vi "Matt-Vibrometer.vi"() -> ()   [LabVIEW 2016]
uses:
  VIs/uPythonX/uPythonX.xctl
panel:
  in  "Tab Control":T1(tab)=enum."Class"
  in  "Vibrometer":T2(xcontrol)={"VISA Refnum in"="ASRL93::INSTR", "Python Code"="import Bars,ssd1327\n\nimport VibSerial\nfrom machine import I2C, Pin\nfrom pyb import ADC  # ADC on machine is limited to under 1.7V\n\ni2c = I2C(2)  # screen\nuart = pyb.UART(1,9600, bits=8, parity=None, stop=1) # vibrometer\ndisplay = ssd1327.SEEED_OLED_96X96(i2c)   # set up display\ndisplay.fill(0)\nlights = Bars.GroveLEDBar('W32','W30',False)\nadc = ADC('X1')\n\n# initialize vibrometer\nsettings = VibSerial.setup(104, 50, True, True)  \nprint(settings)\nSettings = settings.split(', ')\n\n# show settings\ndisplay.text(\"Matt's Box\",0,0,15)\ndisplay.text(' ',0,10,5)\ndisplay.text('HP ' + Settings[0] + 'Hz',0,20,15)\ndisplay.text('BW ' + Settings[1] + 'kHz',0,30,15)\ndisplay.text('S ' + Settings[2] + ' mmps',0,40,15)\ndisplay.show()\n\nwhile True:\n     lights.meter(int(adc.read()/4095*11))\n     utime.sleep(.2)\n     \n"}
  in  "VibSerial":T2(xcontrol)={"VISA Refnum in"="ASRL93::INSTR", "Python Code"="Answer = b'AgAAAAAAAAAAAAAAAAAGAAAAAio=\\n'\n\n#  Laser Toggle\nLaserOn = 'AQAAAAAAAAAAAAAAAAAQAAAAAAAEAgAuAAEAAwEA\\n'\nLaserOff = 'AQAAAAAAAAAAAAAAAAAQAAAAAAAEAgAuAAEAAwAA\\n'\n\n# High Pass Filter\nHighPass_Off = 'AQAAAAAAAAAAAAAAAAAQAAAAAAAEBwAuAgEAAwAA\\n'\nHighPass_13Hz = 'AQAAAAAAAAAAAAAAAAAQAAAAAAAEBwAuAgEAAwEA\\n'\nHighPass_104Hz = 'AQAAAAAAAAAAAAAAAAAQAAAAAAAEBwAuAgEAAwIA\\n'\n\n# Bandwidth\nBandwidth_1kHz = 'AQAAAAAAAAAAAAAAAAAQAAAAAAAEBwASAAEAAwUA\\n'\nBandwidth_5kHz = 'AQAAAAAAAAAAAAAAAAAQAAAAAAAEBwASAAEAAwQA\\n'\nBandwidth_10kHz = 'AQAAAAAAAAAAAAAAAAAQAAAAAAAEBwASAAEAAwMA\\n'\nBandwidth_25kHz = 'AQAAAAAAAAAAAAAAAAAQAAAAAAAEBwASAAEAAwIA\\n'\nBandwidth_50kHz = 'AQAAAAAAAAAAAAAAAAAQAAAAAAAEBwASAAEAAwEA\\n'\nBandwidth_100kHz = 'AQAAAAAAAAAAAAAAAAAQAAAAAAAEBwASAAEAAwAA\\n'\n\n# Sensitivity\nSensitivity_10mmps = 'AQAAAAAAAAAAAAAAAAAQAAAAAAAEBwAKAAEAAwcA\\n'\nSensitivity_20mmps = 'AQAAAAAAAAAAAAAAAAAQAAAAAAAEBwAKAAEAAwYA\\n'\nSensitivity_50mmps = 'AQAAAAAAAAAAAAAAAAAQAAAAAAAEBwAKAAEAAwUA\\n'\nSensitivity_100mmps = 'AQAAAAAAAAAAAAAAAAAQAAAAAAAEBwAKAAEAAwQA\\n'\nSensitivity_200mmps = 'AQAAAAAAAAAAAAAAAAAQAAAAAAAEBwAKAAEAAwMA\\n'\nSensitivity_500mmps = 'AQAAAAAAAAAAAAAAAAAQAAAAAAAEBwAKAAEAAwIA\\n'\nSensitivity_1000mmps = 'AQAAAAAAAAAAAAAAAAAQAAAAAAAEBwAKAAEAAwEA\\n'\nSensitivity_2000mmps = 'AQAAAAAAAAAAAAAAAAAQAAAAAAAEBwAKAAEAAwAA\\n'\n\n# AutoFocus\nFocus = 'AQAAAAAAAAAAAAAAAAAQAAAAAAAEAgBAAAEAAwEA\\n'\n\nlut = {'HP0' : HighPass_Off,'HP13' : HighPass_13Hz,'HP104' : HighPass_104Hz,'BW1' : Bandwidth_1kHz, 'BW5' : Bandwidth_5kHz,'BW10' : Bandwidth_10kHz,'BW25' : Bandwidth_25kHz, 'BW50' : Bandwidth_50kHz, 'BW100' : Bandwidth_100kHz, 'S10' : Sensitivity_10mmps, 'S20' : Sensitivity_20mmps, 'S50' : Sensitivity_50mmps, 'S100' : Sensitivity_100mmps, 'S200' : Sensitivity_200mmps, 'S500' : Sensitivity_500mmps, 'S1000' : Sensitivity_1000mmps, 'S2000' : Sensitivity_2000mmps}\n\ndef Laser(Cmd):  # 0... off, 1... on, 2... focus\n     if (Cmd == 2):\n          vibSet(Focus)\n     elif (Cmd == 1):\n          vibSet(LaserOn)\n     else:\n          vibSet(LaserOff)\n          \ndef vibSet(CmdString):\n     uart.write(CmdString)\n     reply = uart.readline()\n     return (reply == Answer)\n     \ndef PassThrough():\n     if uart.any():\n          uart.readline()  # need more here - need two different serial lines\n          \n\ndef setup(filter=104, bandwidth=50, sensitivity=200, On = True, focus = True):\n\n     reply = ''\n\n     # set high pass filter\n     try:\n          value = lut['HP'+str(filter)]\n     except:\n          value = lut['HP104']\n          filter = 104\n     if vibSet(value):\n          reply = reply + str(filter)\n\n     # set bandwidth\n     try:\n          value = lut['BW'+str(bandwidth)]\n     except:\n          value = lut['BW50']\n          bandwidth = 50\n     if vibSet(value):\n          reply = reply +  ', ' + str(bandwidth)\n\n     # set sensitivity\n     try:\n          value = lut['S'+str(sensitivity)]\n     except:\n          value = lut['S200']\n          sensitivity = 200\n     if vibSet(value):\n          reply = reply +  ', ' + str(sensitivity)\n\n     #turn laser on and autofocus\n     Laser(On)\n     if focus:\n          Laser(2)\n     return reply\n"}
  in  "VibSerial":T2(xcontrol)={"VISA Refnum in"="ASRL93::INSTR", "Python Code"="Answer = b'AgAAAAAAAAAAAAAAAAAGAAAAAio=\\n'\n          \n#  Laser Toggle\nLaserOn = 'AQAAAAAAAAAAAAAAAAAQAAAAAAAEAgAuAAEAAwEA\\n'\nLaserOff = 'AQAAAAAAAAAAAAAAAAAQAAAAAAAEAgAuAAEAAwAA\\n'\n          \n# High Pass Filter\nHighPass_Off = 'AQAAAAAAAAAAAAAAAAAQAAAAAAAEBwAuAgEAAwAA\\n'\nHighPass_13Hz = 'AQAAAAAAAAAAAAAAAAAQAAAAAAAEBwAuAgEAAwEA\\n'\nHighPass_104Hz = 'AQAAAAAAAAAAAAAAAAAQAAAAAAAEBwAuAgEAAwIA\\n'\n          \n# Bandwidth\nBandwidth_1kHz = 'AQAAAAAAAAAAAAAAAAAQAAAAAAAEBwASAAEAAwUA\\n'\nBandwidth_5kHz = 'AQAAAAAAAAAAAAAAAAAQAAAAAAAEBwASAAEAAwQA\\n'\nBandwidth_10kHz = 'AQAAAAAAAAAAAAAAAAAQAAAAAAAEBwASAAEAAwMA\\n'\nBandwidth_25kHz = 'AQAAAAAAAAAAAAAAAAAQAAAAAAAEBwASAAEAAwIA\\n'\nBandwidth_50kHz = 'AQAAAAAAAAAAAAAAAAAQAAAAAAAEBwASAAEAAwEA\\n'\nBandwidth_100kHz = 'AQAAAAAAAAAAAAAAAAAQAAAAAAAEBwASAAEAAwAA\\n'\n          \n# Sensitivity\nSensitivity_10mmps = 'AQAAAAAAAAAAAAAAAAAQAAAAAAAEBwAKAAEAAwcA\\n'\nSensitivity_20mmps = 'AQAAAAAAAAAAAAAAAAAQAAAAAAAEBwAKAAEAAwYA\\n'\nSensitivity_50mmps = 'AQAAAAAAAAAAAAAAAAAQAAAAAAAEBwAKAAEAAwUA\\n'\nSensitivity_100mmps = 'AQAAAAAAAAAAAAAAAAAQAAAAAAAEBwAKAAEAAwQA\\n'\nSensitivity_200mmps = 'AQAAAAAAAAAAAAAAAAAQAAAAAAAEBwAKAAEAAwMA\\n'\nSensitivity_500mmps = 'AQAAAAAAAAAAAAAAAAAQAAAAAAAEBwAKAAEAAwIA\\n'\nSensitivity_1000mmps = 'AQAAAAAAAAAAAAAAAAAQAAAAAAAEBwAKAAEAAwEA\\n'\nSensitivity_2000mmps = 'AQAAAAAAAAAAAAAAAAAQAAAAAAAEBwAKAAEAAwAA\\n'\n          \n# AutoFocus\nFocus = 'AQAAAAAAAAAAAAAAAAAQAAAAAAAEAgBAAAEAAwEA\\n'\n\nclass Vib(object):\n     def __init__(self,UIn,UOut):\n          self.lut = {'HP0' : HighPass_Off,'HP13' : HighPass_13Hz,'HP104' : HighPass_104Hz,'BW1' : Bandwidth_1kHz, 'BW5' : Bandwidth_5kHz,'BW10' : Bandwidth_10kHz,'BW25' : Bandwidth_25kHz, 'BW50' : Bandwidth_50kHz, 'BW100' : Bandwidth_100kHz, 'S10' : Sensitivity_10mmps, 'S20' : Sensitivity_20mmps, 'S50' : Sensitivity_50mmps, 'S100' : Sensitivity_100mmps, 'S200' : Sensitivity_200mmps, 'S500' : Sensitivity_500mmps, 'S1000' : Sensitivity_1000mmps, 'S2000' : Sensitivity_2000mmps}\n          self.uartIN = pyb.UART(UIn,9600, bits=8, parity=None, stop=1) # vibrometer\n          self.uartOUT = pyb.UART(UOut,9600, bits=8, parity=None, stop=1) # vibrometer\n\n     def Laser(self,Cmd):  # 0... off, 1... on, 2... focus\n          if (Cmd == 2):\n               self.vibSet(Focus)\n          elif (Cmd == 1):\n               self.vibSet(LaserOn)\n          else:\n               self.vibSet(LaserOff)\n          \n     def vibSet(self,CmdString):\n          self.uartOUT.write(CmdString)\n          reply = self.uartOUT.readline()\n          return (reply == Answer)\n     \n     def PassThrough(self):\n          if self.uartIN.any():\n               sent = self.uartIN.readline()  # need more here - need two different serial lines\n               seld.uart.OUT.write(sent)\n\n     def setup(self,filter=104, bandwidth=50, sensitivity=200, On = True, focus = True):\n\n          reply = ''\n\n          # set high pass filter\n          try:\n               value = self.lut['HP'+str(filter)]\n          except:\n               value = self.lut['HP104']\n               filter = 104\n          if self.vibSet(value):\n               reply = reply + str(filter)\n\n          # set bandwidth\n          try:\n               value = self.lut['BW'+str(bandwidth)]\n          except:\n               value = self.lut['BW50']\n               bandwidth = 50\n          if self.vibSet(value):\n               reply = reply +  ', ' + str(bandwidth)\n\n          # set sensitivity\n          try:\n               value = self.lut['S'+str(sensitivity)]\n          except:\n               value = self.lut['S200']\n               sensitivity = 200\n          if self.vibSet(value):\n               reply = reply +  ', ' + str(sensitivity)\n\n          #turn laser on and autofocus\n          self.Laser(LaserOn)\n          if focus:\n               self.Laser(2)\n          return reply\n"}
  in  "Bars":T2(xcontrol)={"VISA Refnum in"="ASRL93::INSTR", "Python Code"="'''\nhttp://wiki.seeedstudio.com/Grove-LED_Bar/\nhttps://github.com/Seeed-Studio/Grove_LED_Bar/blob/master/Grove_LED_Bar.cpp\nhttps://github.com/Seeed-Studio/Grove_LED_Bar/blob/master/examples/BasicControl/BasicControl.ino\n\nconnections: \nGround (B) - GND \nPower  (R)   - 3V3 \nDCLK (W) - pin W30\nDIn (Y) -  pin W32\n'''\n\nimport  utime\nfrom machine import Pin\n\nGLB_CMDMODE = 0x00  # Work on 8-bit mode\nMAX_BRIGHTNESS = 0xFF\n\nclass GroveLEDBar(object):\n     def __init__(self, dio,clk,RtoG=True):\n          self.dio = Pin(dio, Pin.OUT,Pin.PULL_UP)\n          self.clk = Pin(clk, Pin.OUT,Pin.PULL_UP)\n          self.RtoG = RtoG\n          self.stateArray = bytearray(10)\n          for i in range(10):\n               self.stateArray[i] = 0x00  # allows me to toggle individual elements\n\n     def sendData(self,data):\n          state = 0\n          for i in range(16):\n               state1 = (data & 0x8000)\n               self.dio.value(state1)\n               state=1-state\n               self.clk.value(state)\n               data<<=1\n          \n     def latchData(self):\n          self.dio.value(0)\n          utime.sleep_ms(10)\n          for i in range(4):\n               self.dio.value(1)\n               utime.sleep_us(1)\n               self.dio.value(0)\n               utime.sleep_us(1)\n          \n     def setData(self):\n          self.sendData(GLB_CMDMODE)\n          for i in range(10):\n               self.sendData(self.stateArray[i])\n               \n          self.sendData(0x00)  \n          self.sendData(0x00)\n          self.latchData()\n          \n     def setBits(self,bits):\n          for  i in range(10):\n               if self.RtoG:\n                    j = i\n               else:\n                    j = 9-i\n               if ((bits % 2) == 1):\n                    self.stateArray[j] = MAX_BRIGHTNESS\n               else:\n                    self.stateArray[j] = 0x00\n               bits = int(bits / 2)\n          self.setData()\n\n     def setBrightness(self,led,brightness):\n          led = min(9,max((led-1),0))\n          brightness = min (1,max(brightness,0))\n          if ~self.RtoG:\n               led = 9-led\n          self.stateArray[led] =0xFF & ~(~0<< int(8*brightness))\n          self.setData()\n\n     def toggleLED(self,led):\n          led = min(9,max((led-1),0))\n          if ~self.RtoG:\n               led = 9-led\n          self.stateArray[led] = ~ self.stateArray[led]\n          self.setData()\n          \n     def meter(self,value):\n          value = min(10,max(value,0))\n          self.setBits(-1 + 2**value)\n"}
  in  "ssd1327":T2(xcontrol)={"VISA Refnum in"="ASRL93::INSTR", "Python Code"="'''\nMicroPython SSD1327 OLED I2C driver\nhttps://github.com/mcauser/micropython-ssd1327\nMIT License\nCopyright (c) 2017 Mike Causer\nPermission is hereby granted, free of charge, to any person obtaining a copy\nof this software and associated documentation files (the \"Software\"), to deal\nin the Software without restriction, including without limitation the rights\nto use, copy, modify, merge, publish, distribute, sublicense, and/or sell\ncopies of the Software, and to permit persons to whom the Software is\nfurnished to do so, subject to the following conditions:\nThe above copyright notice and this permission notice shall be included in all\ncopies or substantial portions of the Software.\nTHE SOFTWARE IS PROVIDED \"AS IS\", WITHOUT WARRANTY OF ANY KIND, EXPRESS OR\nIMPLIED, INCLUDING BUT NOT LIMITED TO THE WARRANTIES OF MERCHANTABILITY,\nFITNESS FOR A PARTICULAR PURPOSE AND NONINFRINGEMENT. IN NO EVENT SHALL THE\nAUTHORS OR COPYRIGHT HOLDERS BE LIABLE FOR ANY CLAIM, DAMAGES OR OTHER\nLIABILITY, WHETHER IN AN ACTION OF CONTRACT, TORT OR OTHERWISE, ARISING FROM,\nOUT OF OR IN CONNECTION WITH THE SOFTWARE OR THE USE OR OTHER DEALINGS IN THE\nSOFTWARE.\n'''\n\nfrom micropython import const\nimport time\nimport framebuf\n\n\n# commands\nSET_COL_ADDR          = const(0x15)\nSET_SCROLL_DEACTIVATE = const(0x2E)\nSET_ROW_ADDR          = const(0x75)\nSET_CONTRAST          = const(0x81)\nSET_SEG_REMAP         = const(0xA0)\nSET_DISP_START_LINE   = const(0xA1)\nSET_DISP_OFFSET       = const(0xA2)\nSET_DISP_MODE         = const(0xA4) # 0xA4 normal, 0xA5 all on, 0xA6 all off, 0xA7 when inverted\nSET_MUX_RATIO         = const(0xA8)\nSET_FN_SELECT_A       = const(0xAB)\nSET_DISP              = const(0xAE) # 0xAE power off, 0xAF power on\nSET_PHASE_LEN         = const(0xB1)\nSET_DISP_CLK_DIV      = const(0xB3)\nSET_SECOND_PRECHARGE  = const(0xB6)\nSET_GRAYSCALE_TABLE   = const(0xB8)\nSET_GRAYSCALE_LINEAR  = const(0xB9)\nSET_PRECHARGE         = const(0xBC)\nSET_VCOM_DESEL        = const(0xBE)\nSET_FN_SELECT_B       = const(0xD5)\nSET_COMMAND_LOCK      = const(0xFD)\n\n# registers\nREG_CMD  = const(0x80)\nREG_DATA = const(0x40)\n\n\nclass SSD1327:\n     def __init__(self, width, height, external_vcc):\n          self.width = width\n          self.height = height\n          self.external_vcc = external_vcc\n          self.buffer = bytearray(self.width * self.height // 2)\n          self.framebuf = framebuf.FrameBuffer(self.buffer, self.width, self.height, framebuf.GS4_HMSB)\n          self.poweron()\n          self.init_display()\n\n     def init_display(self):\n          for cmd in (\n               SET_COMMAND_LOCK, 0x12, # Unlock\n               SET_DISP, # Display off\n               # Resolution and layout\n               SET_DISP_START_LINE, 0x00,\n               SET_DISP_OFFSET, 0x20, # Set vertical offset by COM from 0~127\n               # Set re-map\n               # Enable column address re-map\n               # Disable nibble re-map\n               # Horizontal address increment\n               # Enable COM re-map\n               # Enable COM split odd even\n               SET_SEG_REMAP, 0x51,\n               SET_MUX_RATIO, self.height - 1,\n               # Timing and driving scheme\n               SET_FN_SELECT_A, 0x01, # Enable internal VDD regulator\n               SET_PHASE_LEN, 0x51, # Phase 1: 1 DCLK, Phase 2: 5 DCLKs\n               SET_DISP_CLK_DIV, 0x01, # Divide ratio: 1, Oscillator Frequency: 0\n               SET_PRECHARGE, 0x08, # Set pre-charge voltage level: VCOMH\n               SET_VCOM_DESEL, 0x07, # Set VCOMH COM deselect voltage level: 0.86*Vcc\n               SET_SECOND_PRECHARGE, 0x01, # Second Pre-charge period: 1 DCLK\n               SET_FN_SELECT_B, 0x62, # Enable enternal VSL, Enable second precharge\n               # Display\n               SET_GRAYSCALE_LINEAR, # Use linear greyscale lookup table\n               SET_CONTRAST, 0x7f, # Medium brightness\n               SET_DISP_MODE, # Normal, not inverted\n               # 96x96:\n               # SET_ROW_ADDR, 0 95,\n               # SET_COL_ADDR, 8, 55,\n               # 128x128:\n               # SET_ROW_ADDR, 0 127,\n               # SET_COL_ADDR, 0, 63,\n               SET_ROW_ADDR, 0x00, self.height - 1,\n               SET_COL_ADDR, ((128 - self.width) // 4), 63 - ((128 - self.width) // 4),\n\n               SET_SCROLL_DEACTIVATE,\n               SET_DISP | 0x01): # Display on\n               self.write_cmd(cmd)\n          self.fill(0)\n          self.show()\n\n     def poweroff(self):\n          self.write_cmd(SET_FN_SELECT_A)\n          self.write_cmd(0x00) # Disable internal VDD regulator, to save power\n          self.write_cmd(SET_DISP)\n\n     def poweron(self):\n          self.write_cmd(SET_FN_SELECT_A)\n          self.write_cmd(0x01) # Enable internal VDD regulator\n          self.write_cmd(SET_DISP | 0x01)\n\n     def contrast(self, contrast):\n          self.write_cmd(SET_CONTRAST)\n          self.write_cmd(contrast) # 0-255\n\n     def invert(self, invert):\n          self.write_cmd(SET_DISP_MODE | (invert & 1) << 1 | (invert & 1)) # 0xA4=Normal, 0xA7=Inverted\n\n     def show(self):\n          self.write_cmd(SET_COL_ADDR)\n          self.write_cmd((128 - self.width) // 4)\n          self.write_cmd(63 - ((128 - self.width) // 4))\n          self.write_cmd(SET_ROW_ADDR)\n          self.write_cmd(0x00)\n          self.write_cmd(self.height - 1)\n          self.write_data(self.buffer)\n\n     def fill(self, col):\n          self.framebuf.fill(col)\n\n     def pixel(self, x, y, col):\n          self.framebuf.pixel(x, y, col)\n\n     def scroll(self, dx, dy):\n          self.framebuf.scroll(dx, dy)\n          # software scroll\n\n     def text(self, string, x, y, col=15):\n          self.framebuf.text(string, x, y, col)\n\n\nclass SSD1327_I2C(SSD1327):\n     def __init__(self, width, height, i2c, addr=0x3c, external_vcc=False):\n          self.i2c = i2c\n          self.addr = addr\n          self.temp = bytearray(2)\n          super().__init__(width, height, external_vcc)\n\n     def write_cmd(self, cmd):\n          self.temp[0] = REG_CMD # Co=1, D/C#=0\n          self.temp[1] = cmd\n          self.i2c.writeto(self.addr,self.temp)\n\n     def write_data(self, buf):\n          self.i2c.writeto(self.addr,b'@' + buf)\n\nclass SEEED_OLED_96X96(SSD1327_I2C):\n     def __init__(self, i2c):\n          super().__init__(96, 96, i2c)\n\n     def rotate(self, rotate):\n          self.poweroff()\n          self.write_cmd(SET_DISP_OFFSET)\n          self.write_cmd(0x60 if rotate else 0x20) # 0x20=0 degrees, 0x60=180 degrees\n          self.write_cmd(SET_SEG_REMAP)\n          self.write_cmd(0x42 if rotate else 0x51) # 0x51=0 degrees, 0x42=180 degrees\n          self.poweron()\n\n     def lookup(self, table):\n          # GS0 has no pre-charge and current drive\n          self.write_cmd(SET_GRAYSCALE_TABLE)\n          for i in range(0,15):\n               self.write_cmd(table[i])\n"}
  in  "OldSerial":T2(xcontrol)={"VISA Refnum in"="ASRL44::INSTR", "Python Code"="import time,pyb\n\nuart = pyb. UART(3,9600, bits=8, parity=None, stop=1)\n\n#  Laser Toggle\n\nLaserOn = 'AQAAAAAAAAAAAAAAAAAQAAAAAAAEAgAuAAEAAwEA\\n'\nLaserOff = 'AQAAAAAAAAAAAAAAAAAQAAAAAAAEAgAuAAEAAwAA\\n'\nLaserAnswer = 'AgAAAAAAAAAAAAAAAAAGAAAAAio='\n\ndef LaserOn(on):\n     if on:\n          uart.write(LaserOn)\n     else:\n          uart.write(LaserOff)\n     reply = uart.read(28)\n     return (reply == LaserAnswer)\n\n# High Pass Filter\n\nHP_Off = 'AQAAAAAAAAAAAAAAAAAQAAAAAAAEBwAuAgEAAwAA\\n'\nHP_13Hz = 'AQAAAAAAAAAAAAAAAAAQAAAAAAAEBwAuAgEAAwEA\\n'\nHP_104Hz = 'AQAAAAAAAAAAAAAAAAAQAAAAAAAEBwAuAgEAAwIA\\n'\nHP_Answer = 'AgAAAAAAAAAAAAAAAAAGAAAAAio='\n\ndef HighPass(option = 0):\n     if option ==1:\n          uart.write(HP_13Hz)\n     elif option == 2:\n          uart.write(HP_104Hz)\n     else:\n          uart.write(HP_Off)\n     reply = uart.read(28)\n     return (reply == HP_Answer)\n\n# Bandwidth\n\nBW_1kHz = 'AQAAAAAAAAAAAAAAAAAQAAAAAAAEBwASAAEAAwUA\\n'\nBW_5kHz = 'AQAAAAAAAAAAAAAAAAAQAAAAAAAEBwASAAEAAwQA\\n'\nBW_10kHz = 'AQAAAAAAAAAAAAAAAAAQAAAAAAAEBwASAAEAAwMA\\n'\nBW_25kHz = 'AQAAAAAAAAAAAAAAAAAQAAAAAAAEBwASAAEAAwIA\\n'\nBW_50kHz = 'AQAAAAAAAAAAAAAAAAAQAAAAAAAEBwASAAEAAwEA\\n'\nBW_100kHz = 'AQAAAAAAAAAAAAAAAAAQAAAAAAAEBwASAAEAAwAA\\n'\nBW_Answer = 'AgAAAAAAAAAAAAAAAAAGAAAAAio='\n\ndef SetBW(option = 4):\n     if option ==0:\n          uart.write(BW_1kHz)\n     elif option == 1:\n          uart.write(BW_5kHz)\n     elif option == 2:\n          uart.write(BW_10kHz)\n     elif option == 3:\n          uart.write(BW_25kHz)\n     elif option == 4:\n          uart.write(BW_50kHz)\n     elif option == 5:\n          uart.write(BW_100kHz)\n     else:\n          uart.write(BW_50kHz)\n     reply = uart.read(28)\n     return (reply == BW_Answer)\n\n# Sensitivity\n\nS_10mmps = 'AQAAAAAAAAAAAAAAAAAQAAAAAAAEBwAKAAEAAwcA\\n'\nS_20mmps = 'AQAAAAAAAAAAAAAAAAAQAAAAAAAEBwAKAAEAAwYA\\n'\nS_50mmps = 'AQAAAAAAAAAAAAAAAAAQAAAAAAAEBwAKAAEAAwUA\\n'\nS_100mmps = 'AQAAAAAAAAAAAAAAAAAQAAAAAAAEBwAKAAEAAwQA\\n'\nS_200mmps = 'AQAAAAAAAAAAAAAAAAAQAAAAAAAEBwAKAAEAAwMA\\n'\nS_500mmps = 'AQAAAAAAAAAAAAAAAAAQAAAAAAAEBwAKAAEAAwIA\\n'\nS_1000mmps = 'AQAAAAAAAAAAAAAAAAAQAAAAAAAEBwAKAAEAAwEA\\n'\nS_2000mmps = 'AQAAAAAAAAAAAAAAAAAQAAAAAAAEBwAKAAEAAwAA\\n'\nS_Answer = 'AgAAAAAAAAAAAAAAAAAGAAAAAio='\n\ndef SetBW(option = 4):\n     if option ==0:\n          uart.write(S_10mmps)\n     elif option == 1:\n          uart.write(S_20mmps)\n     elif option == 2:\n          uart.write(S_50mmps)\n     elif option == 3:\n          uart.write(S_100mmps)\n     elif option == 4:\n          uart.write(S_200mmps)\n     elif option == 5:\n          uart.write(S_500mmps)\n     elif option == 6:\n          uart.write(S_1000mmps)\n     elif option == 7:\n          uart.write(S_2000mmps)\n     else:\n          uart.write(S_200mmps)\n     reply = uart.read(28)\n     return (reply == S_Answer)\n\n# AutoFocus\n\nFocus = 'AQAAAAAAAAAAAAAAAAAQAAAAAAAEAgBAAAEAAwEA\\n'\nFocus_Answer = 'AgAAAAAAAAAAAAAAAAAGAAAAAio='\n\ndef Focus():\n      uart.write(Focus)\n     return (reply == Focus_Answer)\n\nwhile(True):\n    time.sleep_ms(100)\n    size = uart.any()\n    if (size > 0):\n        string = uart.read(size)\n        data = int(string[-1])\n        print('Data: %3d' % (data))\n"}
  in  "Old Screen":T2(xcontrol)={"VISA Refnum in"="ASRL44::INSTR", "Python Code"="from machine import I2C, Pin\nimport utime\nimport framebuf\n\ni2c = I2C(2)\n\nOLED_Address = 0x3c\nOLED_Command_Mode = 0x80\nOLED_Data_Mode = 0x40\nOLED_Display_Off_Cmd = 0xAE\nOLED_Display_On_Cmd = 0xAF\nOLED_Normal_Display_Cmd = 0xA4\nOLED_Normal_Display_Cmd_SH1107G = 0xA6\nOLED_Inverse_Display_Cmd = 0xA7\nOLED_Activate_Scroll_Cmd = 0x2F\nOLED_Dectivate_Scroll_Cmd = 0x2E\nOLED_Set_ContrastLevel_Cmd = 0x81\n\n#define frame buffer\nbuffer = bytearray(96*96//2)\nframe = framebuf.FrameBuffer(buffer,96,96,framebuf.GS4_HMSB)\n\n\ndef init_SSD1327():\n     sendCommand(0xFD)  #  Unlock OLED driver IC MCU interface from entering command. i.e: Accept commands\n     sendCommand(0x12)\n     sendCommand(0xAE)  #  Set display off\n     sendCommand(0xA8)  #  set multiplex ratio\n     sendCommand(0x5F)  #  96\n     sendCommand(0xA1)  #   set display start line\n     sendCommand(0x00)\n     sendCommand(0xA2)  #  set display offset\n     sendCommand(0x60)\n     sendCommand(0xA0)  #  set remap\n     sendCommand(0x46)\n     sendCommand(0xAB)  #  set vdd internal\n     sendCommand(0x01)\n     sendCommand(0x81)  #  set contrasr\n     sendCommand(0x53)  #  100 nit\n     sendCommand(0xB1)  #   Set Phase Length\n     sendCommand(0X51)\n     sendCommand(0xB3)  #  Set Display Clock Divide Ratio/Oscillator Frequency\n     sendCommand(0x01)\n     sendCommand(0xB9)\n     sendCommand(0xBC)  #  set pre_charge voltage/VCOMH\n     sendCommand(0x08)  \n     sendCommand(0xBE)  #  set VCOMH\n     sendCommand(0X07)\n     sendCommand(0xB6)  #  Set second pre-charge period\n     sendCommand(0x01)\n     sendCommand(0xD5)  #  enable second precharge and enternal vsl\n     sendCommand(0X62)\n     sendCommand(0xA4)  #  Set Normal Display Mode\n     sendCommand(0x2E)  #  Deactivate Scroll\n     sendCommand(0xAF)  #  Switch on display\n     utime.sleep_ms(100)\n     \n     #/ Row Address\n     sendCommand(0x75)  #  Set Row Address \n     sendCommand(0x00)  #  Start 0\n     sendCommand(0x5f)  #  End 95 \n\n     # Column Address\n     sendCommand(0x15)  #  Set Column Address \n     sendCommand(0x08)  #  Start from 8th Column of driver IC. This is 0th Column for OLED \n     sendCommand(0x37)  #  End at  (8 + 47)th column. Each Column has 2 pixels(segments)\n\n     # Init gray level for text. Default:Brightest White\n     grayH= 0xF0\n     grayL= 0x0F\n     \n     \n     \ndef init_SH1107G():\n     sendCommand(0xae)  # Display OFF \n     sendCommand(0xd5)  # Set Dclk\n     sendCommand(0x50)  # 100Hz\n     sendCommand(0x20)  # Set row address\n     sendCommand(0x81)  # Set contrast control\n     sendCommand(0x80) \n     sendCommand(0xa0)  # Segment remap\n     sendCommand(0xa4)  # Set Entire Display ON \n     sendCommand(0xa6)  # Normal display\n     sendCommand(0xad)  # Set external VCC\n     sendCommand(0x80)\n     sendCommand(0xc0)  # Set Common scan direction\n     sendCommand(0xd9)  # Set phase length\n     sendCommand(0x1f)\n     sendCommand(0xdb)  # Set Vcomh voltage\n     sendCommand(0x27)\n     sendCommand(0xaf)  # Display ON\n     sendCommand(0xb0)\n     sendCommand(0x00)\n     sendCommand(0x11)\n\ndef sendCommand(cmd):\n     temp = bytearray(2)\n     temp[0] = OLED_Command_Mode\n     temp[1] = cmd\n     i2c.writeto(OLED_Address,temp)\n\ndef sendData(data):\n     i2c.writeto(OLED_Address,b'@' + data)\n\ndef clearDisplay():\n     frame.fill(0)\n     sendData(buffer)\n               \ndef fillDisplay():\n     frame.fill(255)\n     sendData(buffer)\n               \ndef partialDisplay():\n     frame.text('Hi there',0,0,15)\n     sendData(buffer)"}
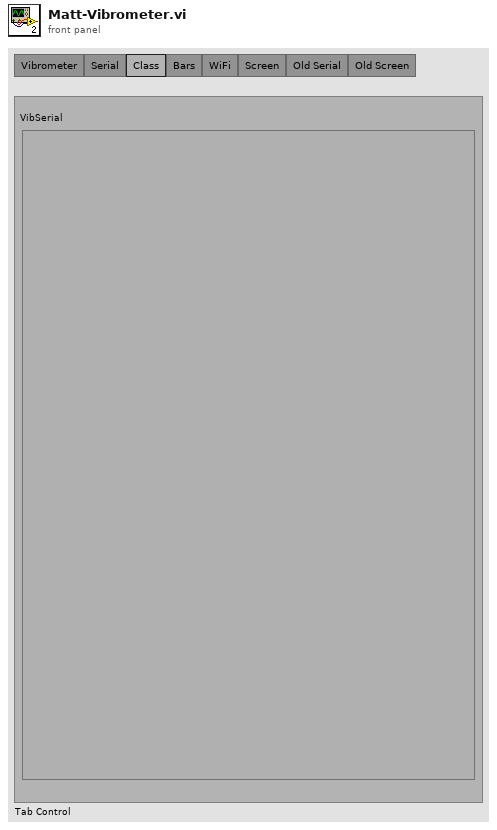
[diagram p1: front panel]
types:
  T1 = enum32{"Vibrometer", "Serial", "Class", "Bars", "WiFi", "Screen", "Old Serial", "Old Screen"}
  T2 = cluster{"VISA Refnum in":refnum<visa-resource-name>, "Python Code":string}
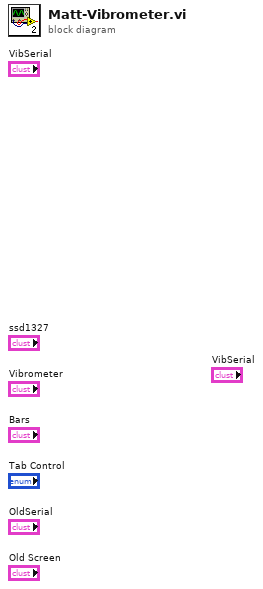
[diagram p0: block diagram]
diagram:
